vi "Stop.vi"(8 "error in (no error)":errorcluster, 11 "Oscilloscope in":refnum<class "Oscilloscope.lvclass">) -> (0 "error out":errorcluster, 3 "Oscilloscope out":refnum<class "Oscilloscope.lvclass">)   [LabVIEW 2015]
uses:
  Oscilloscope.lvclass
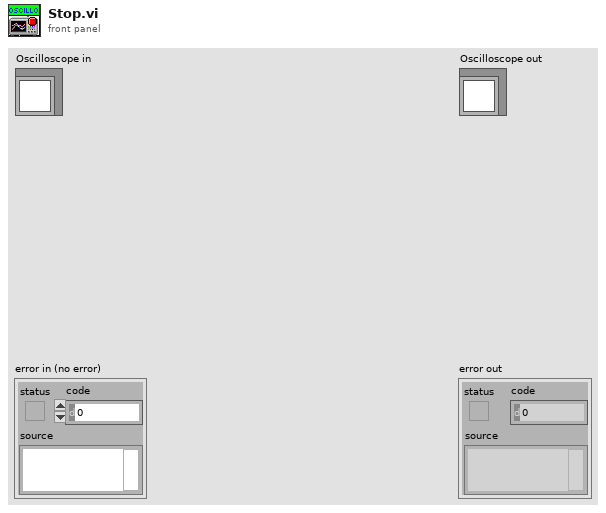
[diagram p1: front panel]
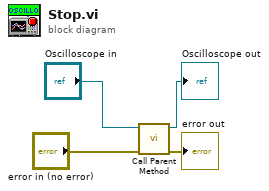
[diagram p0: block diagram]
diagram:
  n1 = call-parent "Call Parent Method"("error in (no error)"="error in (no error)", "Stop in"="Oscilloscope in") -> ("error out"=→"error out":errorcluster, "Stop out"=→"Oscilloscope out":refnum<class "Oscilloscope.lvclass">)  [unwired: 8 in]
